vi "File_type_Excel.vi"() -> ()   [LabVIEW 2011]
panel:
  out "appended path":path
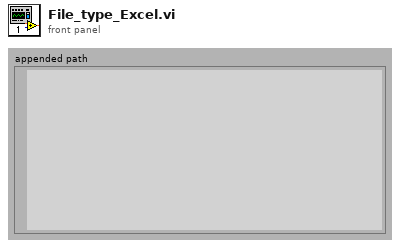
[diagram p1: front panel]
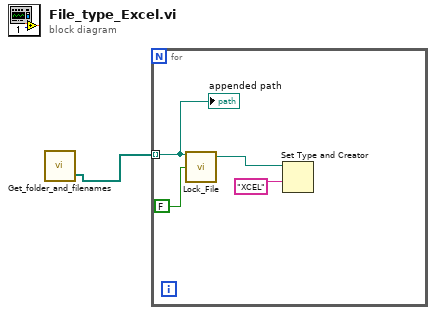
[diagram p0: block diagram]
diagram:
  n1 = call "Get_folder_and_filenames.vi"() -> ("Files"=w1:path[])  [unwired: 1 in, 1 out]
  n2 = for {
    tunnel: w1 -> [w3] mode=indexing
    n3 = call "Lock_File.vi"("Lock File"=FALSE, "path"=w3) -> ("dup path"=w4:path)  [unwired: 2 in, 1 out]
    n4 = Set Type and Creator(5:"XCEL", 7:w4) -> ()  [unwired: 2 in, 2 out]
    "appended path" <- w3
  }
